vi "KeyUnSwitched.vi"(8 "error in (no error)":errorcluster, 9 "Key":T1 {"Time" format="%<%.3X>T"}, 11 "Gviewer in":refnum<class "Gviewer.lvclass">) -> (0 "error out":errorcluster, 3 "Gviewer out":refnum<class "Gviewer.lvclass">)   [LabVIEW 2020, in "Gviewer.lvclass"]
doc: "Andre Koelewijn, 8 jan 2021\n\nIf a switch is pressed then this VI hold the code for the action.\nIf a key stroke combined with another action is used then it is possible that such code resides in another part of the program."
uses:
  Gviewer.lvclass
  controls/KeyPress.ctl
  <vilib>/event_ctls.llb/eventvkey.ctl
  Gviewer.lvclass/Gviewer.ctl
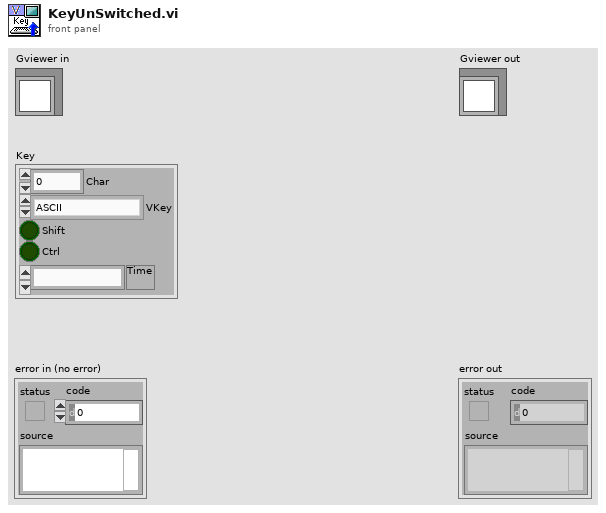
[diagram p1: front panel]
types:
  T1 = typedef "Gviewer.lvclass/KeyPress.ctl" = cluster{"Char":i16, "VKey":T2, "Shift":bool, "Ctrl":bool, "Time":timestamp}
  T2 = typedef "eventvkey.ctl" = enum16{"ASCII", "Enter", "Return", "Shift", "Ctrl", "Alt", "Cmd", "Opt", "Caps", "NumLock", "Clear", "Break", "Up", "Down", "Left", "Right", "Insert", "Delete", "Home", "End", "PageUp", "PageDown", "Escape", "Help", "Pause", "ScrollLock", "F1", "F2", "F3", "F4", "F5", "F6", "F7", "F8", "F9", "F10", "F11", "F12", "F13", "F14", "F15", "F16", "F17", "F18", "F19", "F20", "F21", "F22", "F23", "F24", "Play", "VolumeUp", "VolumeDown", "Mute", "Two Byte Char"}
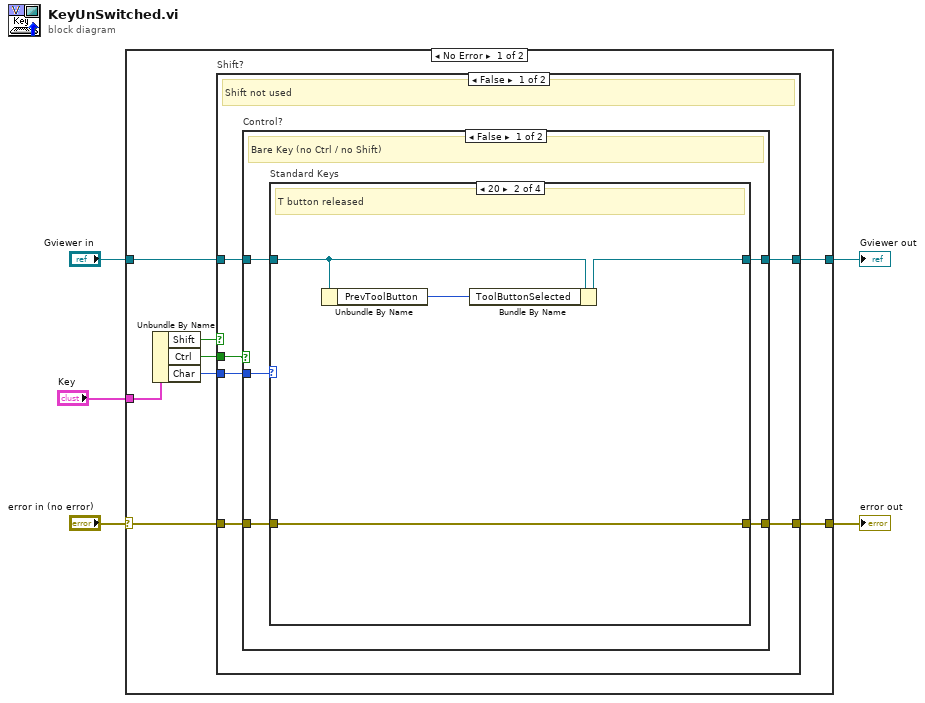
[diagram p0: block diagram]
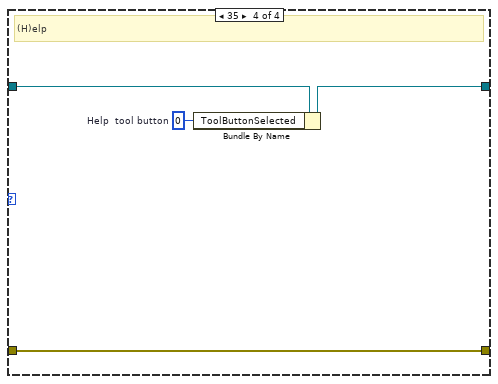
[diagram p4: hidden frame]
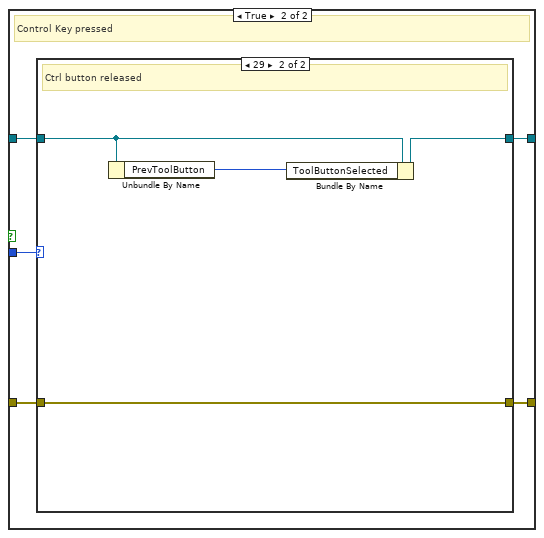
[diagram p5: hidden frame]
diagram:
  n1 = case shown="No Error" "error in (no error)" {
    selector: "error in (no error)" -> [w8 w58]
    tunnel: [w7 w58] -> w4
    tunnel: [w9 w57] -> w2
    tunnel: "Gviewer in" -> [w10 w57]
    tunnel: "Key" -> [w13 _]
    frame No Error {
      n2 = Unbundle By Name(w13) -> ("Shift"=w12:bool, "Ctrl"=w11:bool, "Char"=w6:i16)
      n3 = case "Shift?" shown="False" w12 {
        tunnel: w11 -> [w19 w52]
        tunnel: w10 -> [w18 w51]
        tunnel: [w17 w50] -> w9
        tunnel: w8 -> [w16 w49]
        tunnel: [w15 w48] -> w7
        tunnel: w6 -> [w14 _]
        frame False {
          # "Shift not used"
          n4 = case "Control?" shown="False" w19 {
            tunnel: [w22 w37] -> w17
            tunnel: w18 -> [w23 w40]
            tunnel: [w20 w38] -> w15
            tunnel: w16 -> [w21 w39]
            tunnel: w14 -> [w24 w41]
            frame False {
              # "Bare Key (no Ctrl / no Shift)"
              n5 = case "Standard Keys" shown="20" w24 {
                tunnel: w23 -> [w26 w27 w31 w33]
                tunnel: [w26 w28 w31 w34] -> w22
                tunnel: [w25 w30 w32 w36] -> w20
                tunnel: w21 -> [w25 w30 w32 w36]
                frame Default {
                  # "Not implemented"
                }
                frame 20 {
                  # "T button released"
                  n6 = Unbundle By Name(w27) -> ("PrevToolButton"=w29:i32)
                  n7 = Bundle By Name(cluster=w27, "ToolButtonSelected"=w29) -> (w28:refnum<class "Gviewer.lvclass">)
                }
                frame 1 {
                  # "ESC key"
                }
                frame 35 {
                  w35 = 0  # Help  tool button
                  # "(H)elp"
                  n8 = Bundle By Name(cluster=w33, "ToolButtonSelected"=w35) -> (w34:refnum<class "Gviewer.lvclass">)
                }
              }
            }
            frame True {
              # "Control Key pressed"
              n9 = case shown="29" w41 {
                tunnel: w40 -> [w42 w44]
                tunnel: w39 -> [w43 w47]
                tunnel: [w43 w47] -> w38
                tunnel: [w42 w45] -> w37
                frame Default {
                  # "Not defined"
                }
                frame 29 {
                  # "Ctrl button released"
                  n10 = Unbundle By Name(w44) -> ("PrevToolButton"=w46:i32)
                  n11 = Bundle By Name(cluster=w44, "ToolButtonSelected"=w46) -> (w45:refnum<class "Gviewer.lvclass">)
                }
              }
            }
          }
        }
        frame True {
          # "Shift Pressed"
          n12 = case "Control?" shown="False" w52 {
            tunnel: w51 -> [w54 w56]
            tunnel: [w54 w56] -> w50
            tunnel: w49 -> [w53 w55]
            tunnel: [w53 w55] -> w48
            frame False {
              # "Control Key not pressed: Only Shift Key used"
            }
            frame True {
              # "Control Key Pressed"
            }
          }
        }
      }
    }
    frame Error {
    }
  }
  "error out" <- w4
  "Gviewer out" <- w2
